vi "加标回收数据处理整合 (子VI).vi"(11 "枚举":enum16{"实时数据排序", "小时数据排序"}(ring)) -> (3 "已排序的数组":string[](array[string]))   [LabVIEW 2016, in "数据传输系统-02.lvlib"]
uses:
  <userlib>/_OpenG.lib/array/array.llb/Remove Duplicates from 1D Array (String)__ogtk.vi
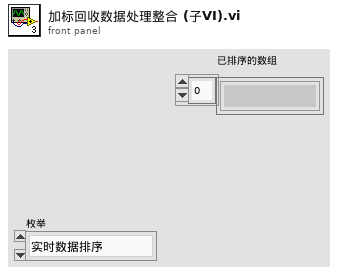
[diagram p1: front panel]
types:
  T1 = cluster{"PH":string[][], "CODCr":string[][], "氨氮":string[][], "CODMn":string[][], "总氮":string[][], "总磷":string[][], "电导率":string[][], "水温":string[][], "DO":string[][], "浊度":string[][], "叶绿素":string[][], "藻密度":string[][], "铜":string[][], "盐度":string[][], "水位":string[][], "流速":string[][], "瞬时流量":string[][], "累积流量":string[][], "亚硝酸盐":string[][], "硫化物":string[][], "ORP":string[][], "铅":string[][], "镉":string[][], "锌":string[][], "镍":string[][], "锰":string[][], "汞":string[][], "气温":string[][], "气压":string[][], "风速":string[][], "风向":string[][], "盐度 2":string[][], "磷酸盐":string[][], "硝氮":string[][], "氟化物":string[][]}
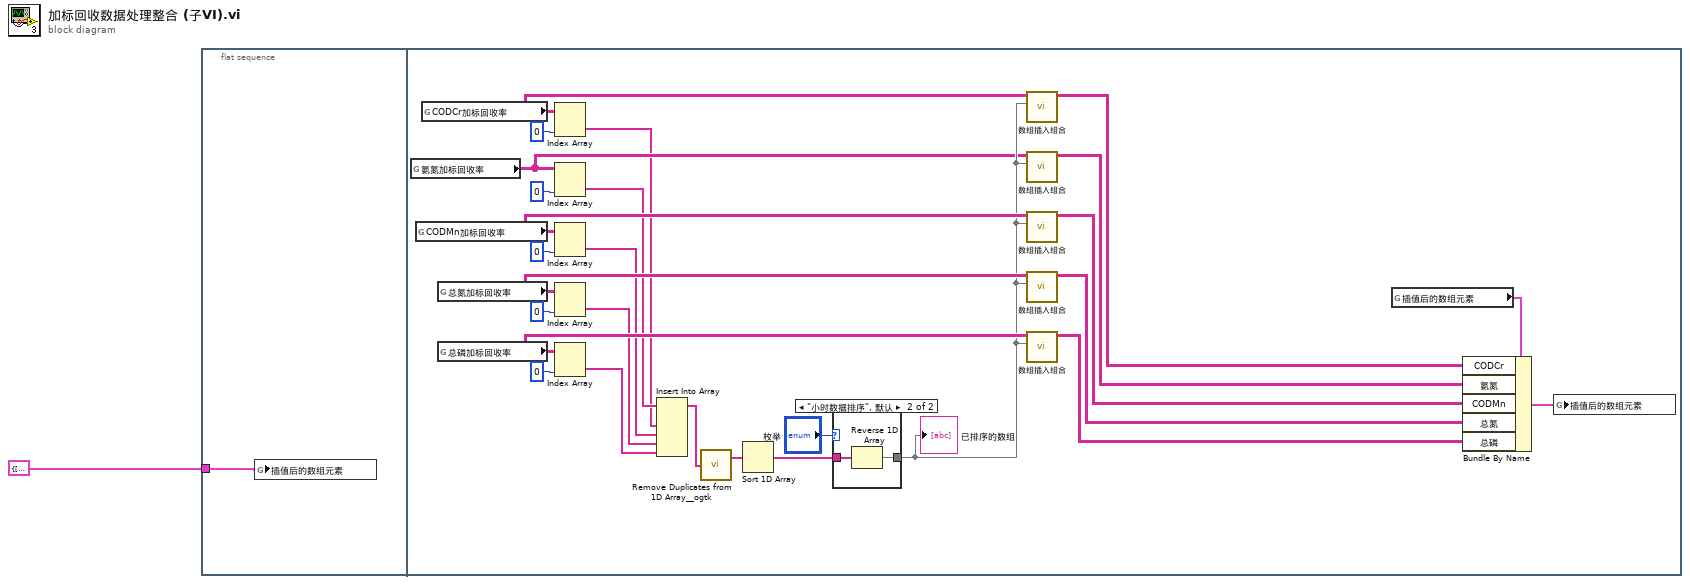
[diagram p0: block diagram]
diagram:
  n1 = flat-sequence {
    tunnel: T1 {"PH"=[], "CODCr"=[], "氨氮"=[], "CODMn"=[], "总氮"=[], "总磷"=[], "电导率"=[], "水温"=[], "DO"=[], "浊度"=[], "叶绿素"=[], "藻密度"=[], "铜"=[], "盐度"=[], "水位"=[], "流速"=[], "瞬时流量"=[], "累积流量"=[], "亚硝酸盐"=[], "硫化物"=[], "ORP"=[], "铅"=[], "镉"=[], "锌"=[], "镍"=[], "锰"=[], "汞"=[], "气温"=[], "气压"=[], "风速"=[], "风向"=[], "盐度 2"=[], "磷酸盐"=[], "硝氮"=[], "氟化物"=[]} ("插值后的数组元素") -> [w2]
    frame #0 {
      n2 = global write "插值后的新数组.vi" "插值后的数组元素"(w2) -> ()
    }
    frame #1 {
      n3 = global read "全局 所有参数.vi" "氨氮加标回收率"() -> (w10:string[][])
      n4 = global read "全局 所有参数.vi" "CODMn加标回收率"() -> (w22:string[][])
      n5 = global read "全局 所有参数.vi" "CODCr加标回收率"() -> (w21:string[][])
      n6 = global read "全局 所有参数.vi" "总氮加标回收率"() -> (w23:string[][])
      n7 = global read "全局 所有参数.vi" "总磷加标回收率"() -> (w24:string[][])
      n8 = Index Array(array=w21, index (col)=0 ("索引 (行)")) -> (element=w8:string[])  [unwired: 1 in]
      n9 = Index Array(array=w10, index (col)=0 ("索引 (行)")) -> (element=w9:string[])  [unwired: 1 in]
      n10 = Index Array(array=w22, index (col)=0 ("索引 (行)")) -> (element=w7:string[])  [unwired: 1 in]
      n11 = Index Array(array=w23, index (col)=0 ("索引 (行)")) -> (element=w6:string[])  [unwired: 1 in]
      n12 = Index Array(array=w24, index (col)=0 ("索引 (行)")) -> (element=w5:string[])  [unwired: 1 in]
      n13 = Insert Into Array(array=w9, new element #1=w8, new element #2=w7, new element #3=w6, new element #4=w5) -> (w20:string[])  [unwired: 1 in]
      n14 = call-poly <userlib>:"Remove Duplicates from 1D Array__ogtk.vi"("Input Array"=w20) -> ("Output Array"=w19:string[])  [unwired: 1 out]
      n15 = Sort 1D Array(array=w19) -> (sorted array=w12:string[])
      n16 = case shown="\"小时数据排序\", 默认" "枚举" {
        tunnel: w12 -> [w30 w32]
        tunnel: [w30 w31] -> w11
        frame "实时数据排序" {
        }
        frame "小时数据排序", Default {
          n17 = Reverse 1D Array(array=w32) -> (reversed array=w31:string[])
        }
      }
      "已排序的数组" <- w11
      n18 = call "数组插入组合.vi"("排序后的一维数组"=w11, "输入数组"=w21) -> ("输出结果"=w25:string[][])  [unwired: 9 in]
      n19 = call "数组插入组合.vi"("排序后的一维数组"=w11, "输入数组"=w10) -> ("输出结果"=w26:string[][])  [unwired: 9 in]
      n20 = call "数组插入组合.vi"("排序后的一维数组"=w11, "输入数组"=w22) -> ("输出结果"=w27:string[][])  [unwired: 9 in]
      n21 = call "数组插入组合.vi"("排序后的一维数组"=w11, "输入数组"=w23) -> ("输出结果"=w28:string[][])  [unwired: 9 in]
      n22 = call "数组插入组合.vi"("排序后的一维数组"=w11, "输入数组"=w24) -> ("输出结果"=w29:string[][])  [unwired: 9 in]
      n23 = global read "插值后的新数组.vi" "插值后的数组元素"() -> (w4:T1)
      n24 = Bundle By Name(cluster=w4, "CODCr"=w25, "氨氮"=w26, "CODMn"=w27, "总氮"=w28, "总磷"=w29) -> (w3:T1)
      n25 = global write "插值后的新数组.vi" "插值后的数组元素"(w3) -> ()
    }
  }
